vi "Acknowledgement.vi"(0 "Destination Address":u8, 5 "Source Address":u8=27, 7 "PGN":u32, 9 "Control Byte":enum8{"ACK", "NACK", "Access Denied"}(ring), 11 "Group Function":u8) -> (4 "Arb ID":u32 format="%.0x", 8 "Data":u8[](array[numeric]))   [LabVIEW 2023, in "J1939 Utilities.lvlib"]
uses:
  J1939 Utilities.lvlib
  Types/PGN Fields Cluster.ctl
  Convert J1939 ID to CAN Arb ID.vi
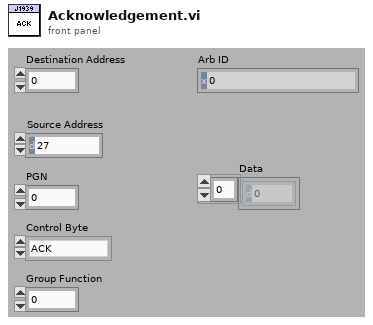
[diagram p1: front panel]
types:
  T1 = typedef "J1939 Utilities.lvlib/PGN Fields Cluster.ctl" = cluster{"Reserved Bit":u8, "Data page":u8, "PDU Format":u8, "PDU Specific":u8}
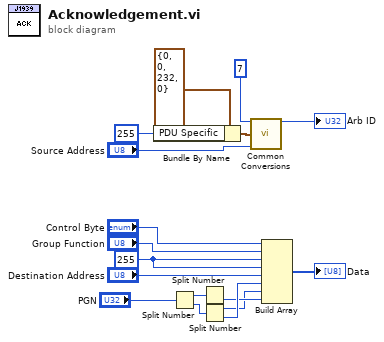
[diagram p0: block diagram]
diagram:
  w11 = u8 255 ("lo")
  n1 = Bundle By Name(cluster=T1 {"Reserved Bit"=0, "Data page"=0, "PDU Format"=232, "PDU Specific"=0} ("PGN Fields"), "PDU Specific"=u8 255) -> (w15:T1)
  n2 = Split Number(x="PGN") -> (hi(x)=w10:u16, lo(x)=w9:u16)
  n3 = Split Number(x=w10) -> (lo(x)=w6:u8)  [unwired: 1 out]
  n4 = Split Number(x=w9) -> (hi(x)=w5:u8, lo(x)=w7:u8)
  n5 = call-poly "Common Conversions.vi"("Priority"=u8 7, "PGN Fields"=w15, "Source Address"="Source Address") -> ("ID"=→"Arb ID":u32)  [unwired: 2 in, 10 out]
  n6 = Build Array("Control Byte", "Group Function", w11, w11, "Destination Address", w7, w5, w6) -> (→"Data":u8[])
